vi "Hardware In - NI 9752-1 (ADCombo).vi"(11 "FPGA Ref":T1) -> (3 "ADCombo":T2)   [LabVIEW 2015, in "ECS-RT.lvlib"]
uses:
  ECS-RT.lvlib
  Typedefs/Raw Inputs/NI9752.ctl
  Typedefs/Raw Inputs/PPWData.ctl
  Typedefs/FPGA Refs/Generic FPGA Ref.ctl
  <vilib>/Utility/error.llb/Error Cluster From Error Code.vi
  <vilib>/rvi/errors/niLvFpgaAdjustHostInterfaceError.vi
  <vilib>/rvi/interface/nirviReadWriteControl/nirviReadWriteControl.xnode
  ECS-Shared.lvlib
  <vilib>/rvi/interface/Simulation/niFpgaSimulationCallBeginRW.vi
  NiFpgaLv.dll
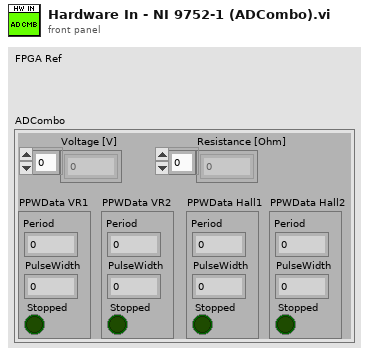
[diagram p1: front panel]
types:
  T1 = typedef "ECS-Shared.lvlib/Generic FPGA Ref.ctl" = refnum<k20>
  T2 = typedef "ECS-Shared.lvlib/NI9752.ctl" = cluster{"Voltage [V]":sgl[], "Resistance [Ohm]":sgl[], "PPWData VR1":T3, "PPWData VR2":T3, "PPWData Hall1":T3, "PPWData Hall2":T3}
  T3 = typedef "ECS-Shared.lvlib/PPWData.ctl" = cluster{"Period":u32, "PulseWidth":u32, "Stopped":bool}
  T4 = cluster{"Result_1":u16, "Result_2":u16, "Result_3":u16, "Result_4":u16, "Result_5":u16, "Result_6":u16, "Result_7":u16, "Result_8":u16, "Result_9":u16, "Result_10":u16, "Result_11":u16, "Result_12":u16, "Result_13":u16, "Result_14":u16, "Result_15":u16, "Result_16":u16, "Result_17":u16, "Result_18":u16, "Result_19":u16, "Result_20":u16, "Result_21":u16, "VRef (2.5V, 0.2%)":u16}
  T5 = cluster{"Period":u32, "PulseWidth":u32, "Stopped":bool}
  T6 = cluster{"Period":u32, "PulseWidth":u32, "Stopped":bool}[]
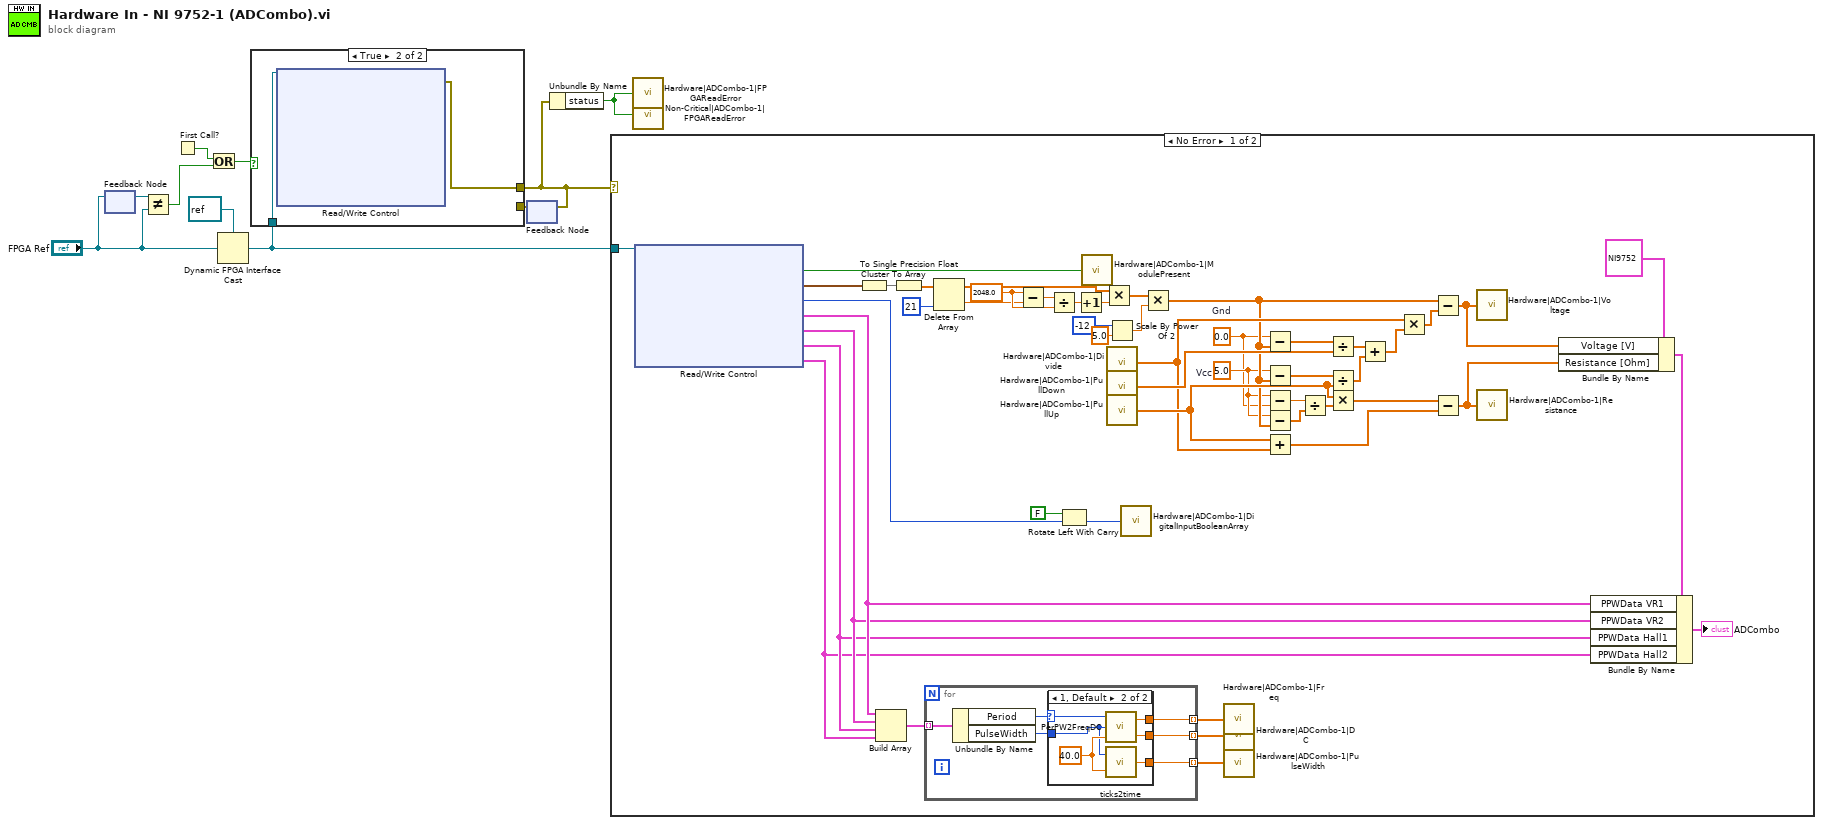
[diagram p0: block diagram]
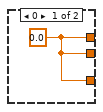
[diagram p3: hidden frame]
diagram:
  n1 = feedback #1() -> (w9:T1)  [unwired: 1 in]
  n2 = feedback-in #1("FPGA Ref") -> ()
  n3 = Not Equal?(x=w9, y="FPGA Ref") -> (x != y?=w10:bool)
  n4 = First Call?() -> (First Call?: T/F=w8:bool)
  n5 = Or(x=w8, y=w10) -> (x .or. y?=w7:bool)
  n6 = Dynamic FPGA Interface Cast(Session In=refnum<k20> refnum ("FPGA VI Reference Out"), Type="FPGA Ref") -> (Session Out=w3:refnum<k20>)
  n7 = feedback #2() -> (w6:errorcluster)  [unwired: 1 in]
  n8 = case shown="True" w7 {
    tunnel: [w11 w13] -> w2
    tunnel: w6 -> [w11 _]
    tunnel: w3 -> [_ w12]
    frame False {
    }
    frame True {
      n9 = xnode "Read/Write Control"("FPGA VI Reference In"=w12) -> ("error out"=w13:errorcluster)  [unwired: 1 in, 9 out]
    }
  }
  n10 = feedback-in #2(w2) -> ()
  n11 = Unbundle By Name(w2) -> ("status"=w1:bool)
  n12 = case shown="No Error" w2 {
    tunnel: w3 -> [w17 _]
    frame No Error {
      w51 = sgl 0.0  # Gnd
      w54 = sgl 5.0  # Vcc
      w40 = sgl 2048.0 ("x")
      n13 = xnode "Read/Write Control"("FPGA VI Reference In"=w17) -> ("ADCombo-1.ModulePresent"=w31:bool, "ADCombo-1.AnalogData"=w32:T4, "ADCombo-1.DigitalTriggers"=w16:u32, "ADCombo-1.VR1.PPWData"=w22:T5, "ADCombo-1.VR2.PPWData"=w21:T5, "ADCombo-1.Hall1.PPWData"=w20:T5, "ADCombo-1.Hall2.PPWData"=w19:T5)  [unwired: 1 in, 2 out]
      n14 = Cluster To Array(cluster=w32) -> (array=w33:u16[])
      n15 = Build Array(w22, w21, w20, w19) -> (w24:T6)
      n16 = To Single Precision Float(number=w33) -> (single precision float=w34:sgl[])
      n17 = for {
        tunnel: w24 -> [w67] mode=indexing
        tunnel: [w64] -> w27 mode=indexing
        tunnel: [w65] -> w26 mode=indexing
        tunnel: [w66] -> w25 mode=indexing
        n18 = Unbundle By Name(w67) -> ("Period"=w63:u32, "PulseWidth"=w68:u32)
        n19 = case shown="1, Default" w63 {
          selector: w63 -> [_ w70]
          tunnel: w68 -> [_ w74]
          tunnel: [w69 w73] -> w66
          tunnel: [w69 w72] -> w65
          tunnel: [w69 w71] -> w64
          frame 0 {
            w69 = sgl 0.0 ("Frequency(Hz)")
          }
          frame 1, Default {
            w75 = sgl 40.0 ("Clock Frequency (MHz, 40)")
            n20 = call <vilib>:"PerPW2FreqDC.vi"("Clock Frequency (MHz, 40)"=w75, "PulseWidth(ticks)"=w74, "Period(ticks)"=w70) -> ("DutyCycle(%)"=w72:sgl, "Frequency(Hz)"=w71:sgl)
            n21 = call <vilib>:"ticks2time.vi"("Clock Frequency (MHz, 40)"=w75, "Ticks"=w74) -> ("Time (msec)"=w73:sgl)
          }
        }
      }
      n22 = Delete From Array(array=w34, index=21) -> (deleted portion=w38:sgl, array with subset deleted=w41:sgl[])  [unwired: 1 in]
      n23 = Subtract(x=w40, y=w38) -> (x-y=w39:sgl)
      n24 = Divide(x=w39, y=w40) -> (x/y=w36:sgl)
      n25 = Rotate Left With Carry(2:w16, 3:FALSE ("carry")) -> (0:w15:u32)  [unwired: 1 out]
      n26 = Increment(x=w36) -> (x+1=w37:sgl)
      n27 = call "Hardware|ADCombo-1|ModulePresent"("Value"=w31) -> ()
      n28 = Multiply(x=w41, y=w37) -> (x*y=w44:sgl[])
      n29 = Scale By Power Of 2(n=i16 -12, x=sgl 5.0) -> (x*2^n=w45:sgl)
      n30 = call "Hardware|ADCombo-1|Divide"() -> ("Value"=w60:sgl[])
      n31 = call "Hardware|ADCombo-1|PullDown"() -> ("Value"=w61:sgl[])
      n32 = call "Hardware|ADCombo-1|PullUp"() -> ("Value"=w62:sgl[])
      n33 = call "Hardware|ADCombo-1|DigitalInputBooleanArray"("Value"=w15) -> ()
      n34 = Multiply(x=w44, y=w45) -> (x*y=w59:sgl[])
      n35 = call "Hardware|ADCombo-1|Freq"("Value"=w27) -> ()
      n36 = call "Hardware|ADCombo-1|DC"("Value"=w26) -> ()
      n37 = call "Hardware|ADCombo-1|PulseWidth"("Value"=w25) -> ()
      n38 = Subtract(x=w51, y=w59) -> (x-y=w48:sgl[])
      n39 = Subtract(x=w54, y=w59) -> (x-y=w47:sgl[])
      n40 = Subtract(x=w54, y=w51) -> (x-y=w52:sgl)
      n41 = Subtract(x=w54, y=w59) -> (x-y=w53:sgl[])
      n42 = Add(x=w62, y=w60) -> (x+y=w58:sgl[])
      n43 = Divide(x=w52, y=w53) -> (x/y=w55:sgl[])
      n44 = Divide(x=w48, y=w61) -> (x/y=w49:sgl[])
      n45 = Divide(x=w47, y=w62) -> (x/y=w56:sgl[])
      n46 = Multiply(x=w62, y=w55) -> (x*y=w57:sgl[])
      n47 = Add(x=w49, y=w56) -> (x+y=w50:sgl[])
      n48 = Multiply(x=w60, y=w50) -> (x*y=w46:sgl[])
      n49 = Subtract(x=w59, y=w46) -> (x-y=w29:sgl[])
      n50 = Subtract(x=w57, y=w58) -> (x-y=w28:sgl[])
      n51 = call "Hardware|ADCombo-1|Voltage"("Value"=w29) -> ()
      n52 = call "Hardware|ADCombo-1|Resistance"("Value"=w28) -> ()
      n53 = Bundle By Name(cluster=T2 {"Voltage [V]"=[], "Resistance [Ohm]"=[], "PPWData VR1"={"Period"=0, "PulseWidth"=0, "Stopped"=FALSE}, "PPWData VR2"={"Period"=0, "PulseWidth"=0, "Stopped"=FALSE}, "PPWData Hall1"={"Period"=0, "PulseWidth"=0, "Stopped"=FALSE}, "PPWData Hall2"={"Period"=0, "PulseWidth"=0, "Stopped"=FALSE}} ("ADCombo"), "Voltage [V]"=w29, "Resistance [Ohm]"=w28) -> (w23:T2)
      n54 = Bundle By Name(cluster=w23, "PPWData VR1"=w22, "PPWData VR2"=w21, "PPWData Hall1"=w20, "PPWData Hall2"=w19) -> (→"ADCombo":T2)
    }
    frame Error {
    }
  }
  n55 = call "Hardware|ADCombo-1|FPGAReadError"("Value"=w1) -> ()
  n56 = call "Non-Critical|ADCombo-1|FPGAReadError"("Fault"=w1) -> ()  [unwired: 2 in]
